vi "Lecroy_wait_OPC-check.vi"(8 "error out":errorcluster, 9 "Start":refnum<vi>, 10 "stop 2":refnum<vi>, 11 "VISA resource name out":refnum<visa-resource-name>) -> (0 "error out 2":errorcluster, 3 "VISA resource name out 2":refnum<visa-resource-name>)   [LabVIEW 2010]
uses:
  <instrlib>/LeCroy Wave Series/LeCroy Wave Series.lvlib
panel:
  in  "stop":bool
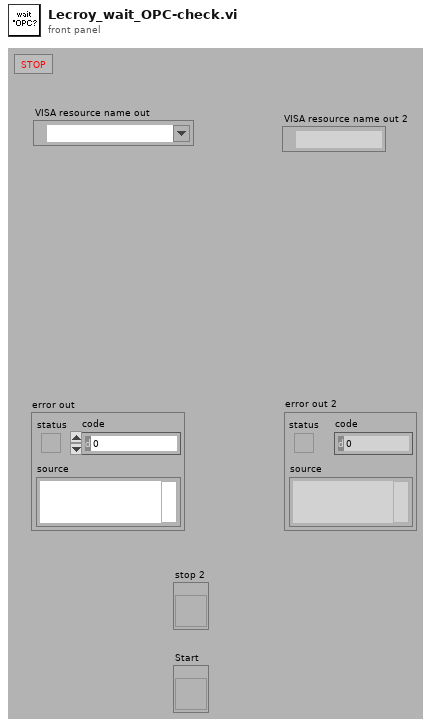
[diagram p1: front panel]
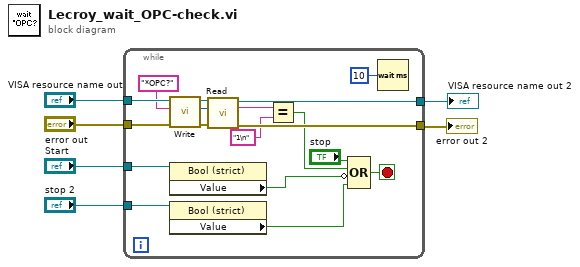
[diagram p0: block diagram]
diagram:
  n1 = while {
    tunnel: "error out" -> [w24]
    tunnel: "VISA resource name out" -> [w23]
    tunnel: [w19] -> w4
    tunnel: [w18] -> w3
    tunnel: "stop 2" -> [w12]
    tunnel: "Start" -> [w11]
    stop <- w14 stop-if-true
    n2 = call <instrlib>:"Write.vi"("error in (no error)"=w24, "Write Buffer"="*OPC?", "VISA resource name"=w23) -> ("error out"=w22:errorcluster, "Return Count"=w21:u32, "VISA resource name out"=w20:refnum<visa-resource-name>)  [unwired: 6 out]
    n3 = property class="Bool (strict)"(reference=w11) -> ("Value"=w10:bool)  [unwired: 1 in, 2 out]
    n4 = property class="Bool (strict)"(reference=w12) -> ("Value"=w9:bool)  [unwired: 1 in, 2 out]
    n5 = call <instrlib>:"Read.vi"("error in (no error)"=w22, "Byte Count"=w21, "VISA resource name"=w20) -> ("error out"=w18:errorcluster, "Read Buffer"=w7:string, "VISA resource name out"=w19:refnum<visa-resource-name>)  [unwired: 6 out]
    n6 = Equal?(x=w7, y="1\n") -> (x = y?=w13:bool)
    n7 = Compound Arithmetic op=OR("stop", w13, invert w10, w9) -> (w14:bool)
    n8 = Wait (ms)(milliseconds to wait=u32 10) -> ()  [unwired: 1 out]
  }
  "VISA resource name out 2" <- w4
  "error out 2" <- w3
